vi "Sequence Execution.vi"() -> ()   [LabVIEW 2013, in "Simple Sequence Tools - Execution.lvlib"]
uses:
  Simple Sequence Tools - Execution.lvlib
  Types/Execute.PreviewMode.ctl
  Types/Execuction.StateVariables.ctl
  Types/Execute.UserEventRefs.ctl
  <vilib>/NI Veristand/Execution/Workspace/SystemStateRegEventRef.ctl
  Types/Execution.SequenceState.ctl
  <vilib>/NI Veristand/Execution/DataLogging/DataLoggingSpecification Ref.ctl
  <vilib>/NI Veristand/Execution/DataLogging/IDataLogging Ref.ctl
  <vilib>/NI Veristand/Execution/Workspace/WorkspaceAPI.ctl
  <vilib>/NI Veristand/Execution/Workspace/SystemStateEventRef.ctl
  Shared/Types/INI.Settings
  NationalInstruments.VeriStand.RealTimeSequenceDefinitionApi
  <vilib>/NI Veristand/Execution/Workspace/NI VeriStand - Set Single Channel Value.vi
  <vilib>/NI Veristand/Execution/Workspace/NI_VS Workspace ExecutionAPI.lvlib
  NationalInstruments.VeriStand.ClientAPI
  Shared/Simple Sequence Tools - Shared.lvlib
  <vilib>/NI Veristand/Execution/DataLogging/NI_VS Data Logging API.lvlib
panel:
  out "Total Iterations":u32=1 min=1 max=2
  out "Current Step":u32 min=1 max=5
  out "Current Iteration":u32=1 min=1 max=2
  in  "NIVS.Gateway IP Address":string="localhost"
  in  "NIVS.Workspace Event":refnum<event-registration>
  in  "Preview Mode":T1=enum."Table"
  in  "Start Step":u32 min=1 max=5
  in  "Start Iteration":u32=1 min=1 max=2
  in  "Log Channels":T2(ring)
  in  "Base File Name":string caption="Base File Name (timestamp included automatically)"
  in  "Enable Logging":bool
  in  "Abort":bool
  in  "Pause":bool
  in  "Start":bool
  in  "Profiles":string(combo)
  out "Graph":waveform(dbl)[](graph)
  out "Sequence":i32[](listbox)
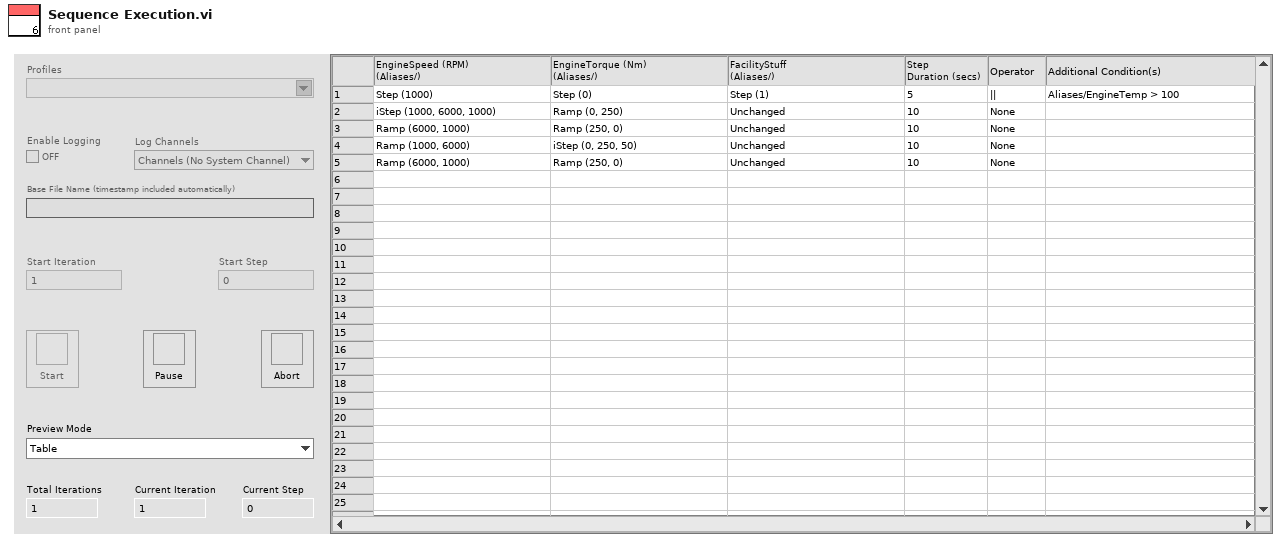
[diagram p1: front panel]
types:
  T1 = typedef "Simple Sequence Tools - Execution.lvlib/Execute.PreviewMode.ctl" = enum8{"Graph", "Table"}
  T2 = enum16{"Channels (No System Channel)", "Aliases", "All"}
  T3 = typedef "Simple Sequence Tools - Execution.lvlib/Execution.SequenceState.ctl" = enum16{"Idle", "Initializing", "Running", "Paused", "Finalizing", "Complete"}
  T4 = typedef "Simple Sequence Tools - Execution.lvlib/Execuction.StateVariables.ctl" = cluster{"NIVS.BaseLogPath":path, "NIVS.SystemDefinitionFile":path, "NIVS.Events":T5, "NIVS.SequenceState":T3, "NIVS.GatewayIPAddress":string, "NIVS.DataLogSpecRef":T7, "NIVS.DataLogManagerRef":T8, "NIVS.LogSessionGUID":string, "NIVS.WorkspaceManager":T9, "NIVS.Deployed":bool, "NIVS.ProfileRef":refnum<k24>, "NIVS.ProfileCallback":refnum<k27>, "NIVS.SystemStateRefs":T10, "UI.Abort":refnum<vi>, "UI.Pause":refnum<vi>, "UI.EnableLogging":refnum<vi>, "UI.Start":refnum<vi>, "UI.LogChannels":refnum<vi>, "UI.StartIteration":refnum<vi>, "UI.StartStep":refnum<vi>, "UI.Sequence":refnum<vi>, "UI.PreviewMode":refnum<vi>, "UI.Graph":refnum<vi>, "UI.BaseFileName":refnum<vi>, "UI.Profiles":refnum<vi>, "UI.CurrentStep":refnum<vi>, "UI.CurrentIteration":refnum<vi>, "UI.TotalIterations":refnum<vi>, "Sequence.AbortChannel":string, "Sequence.StepInfoChannel":string, "Sequence.Iterations":u32, "Sequence.IterationInfoChannel":string, "Sequence.#ofColumns":i32, "Events.State":refnum<user-event>, "Events.Test Result":refnum<user-event>, "Events.Progress":refnum<user-event>, "INI.Settings":T11}
  T5 = typedef "Simple Sequence Tools - Execution.lvlib/Execute.UserEventRefs.ctl" = cluster{"SequenceEvent":refnum<event-registration>, "SystemChangeEvent":T6, "WorkspaceEvent":refnum<event-registration>}
  T6 = typedef "NI_VS Workspace ExecutionAPI.lvlib/SystemStateRegEventRef.ctl" = refnum<event-registration>
  T7 = typedef "NI_VS Data Logging API.lvlib/DataLoggingSpecification Ref.ctl" = refnum<k24>
  T8 = typedef "NI_VS Data Logging API.lvlib/IDataLogging Ref.ctl" = refnum<k24>
  T9 = typedef "NI_VS Workspace ExecutionAPI.lvlib/WorkspaceAPI.ctl" = refnum<k24>
  T10 = typedef "NI_VS Workspace ExecutionAPI.lvlib/SystemStateEventRef.ctl" = cluster{"CustDatRef":refnum<user-event>, "EvtRef":refnum<k27>}
  T11 = typedef "Simple Sequence Tools - Shared.lvlib/INI.Settings" = cluster{"Build Location":path, "LoggingLocation":path}
  T12 = enum8{"Enabled", "Disabled", "Disabled and Grayed Out"}
  T13 = typedef "NI_VS Workspace ExecutionAPI.lvlib/SystemState.ctl" = u8
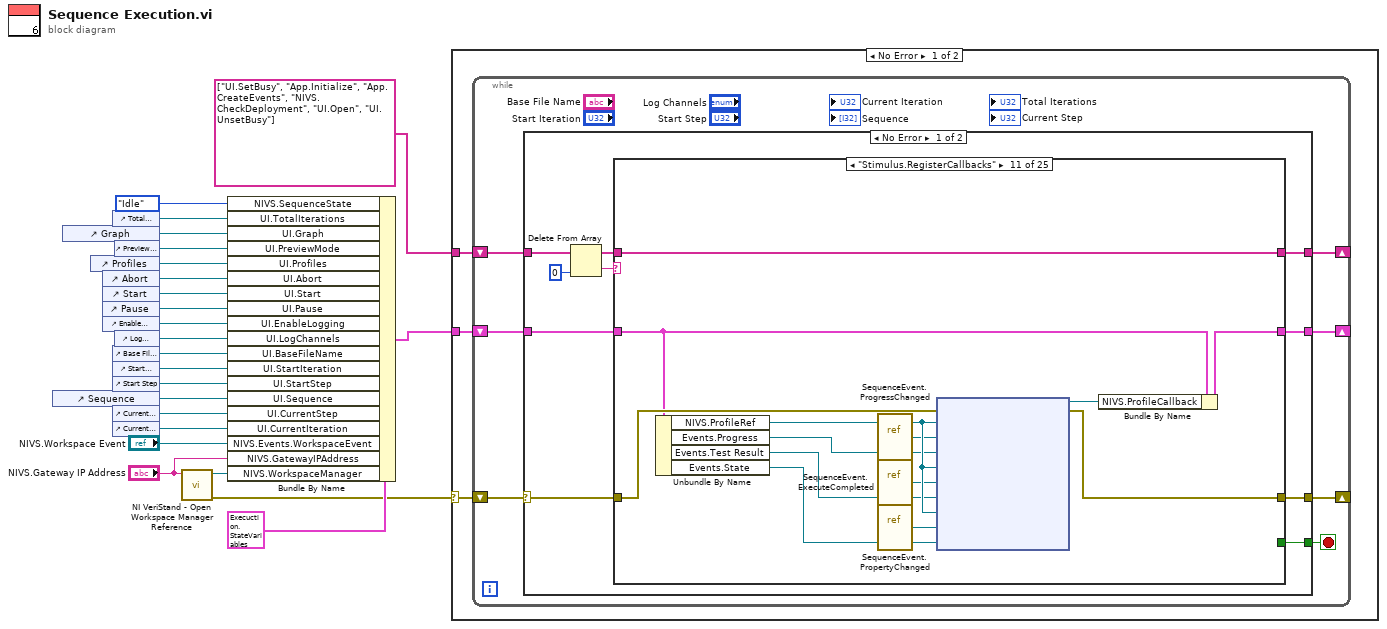
[diagram p0: block diagram]
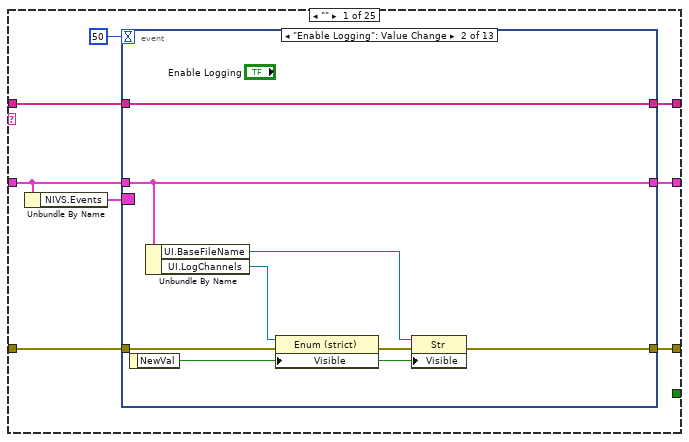
[diagram p2: hidden frame]
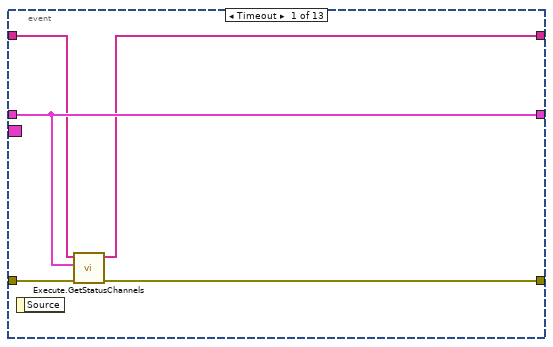
[diagram p3: hidden frame]
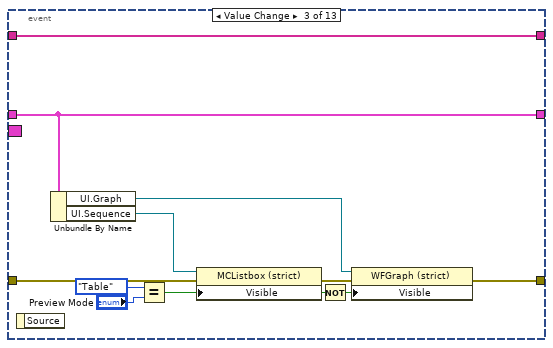
[diagram p4: hidden frame]
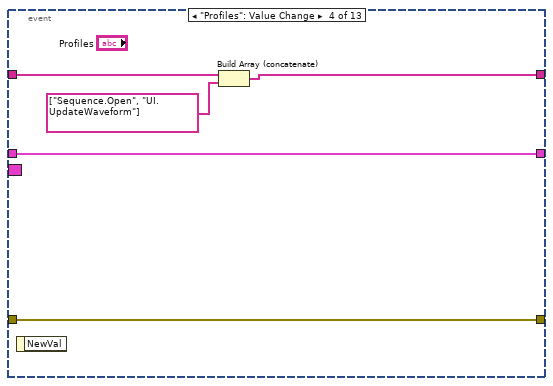
[diagram p5: hidden frame]
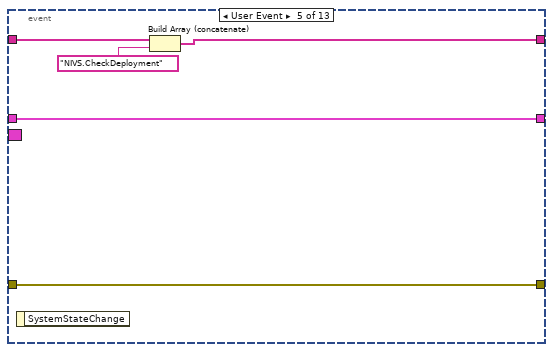
[diagram p6: hidden frame]
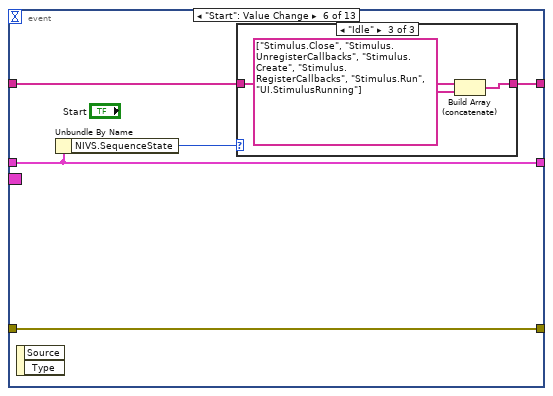
[diagram p7: hidden frame]
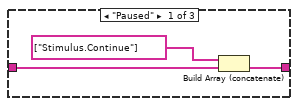
[diagram p8: hidden frame]
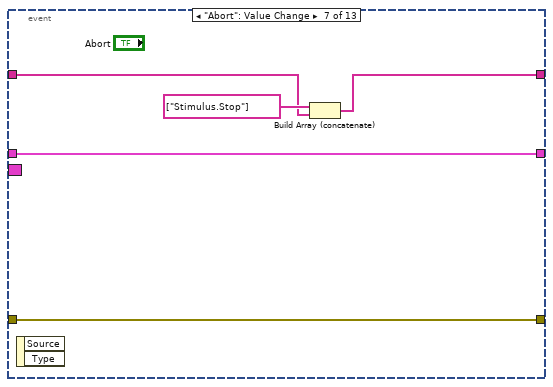
[diagram p10: hidden frame]
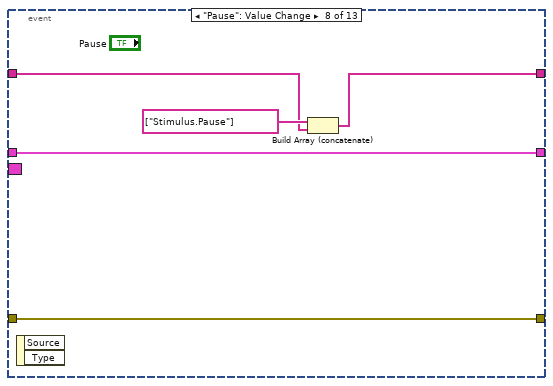
[diagram p11: hidden frame]
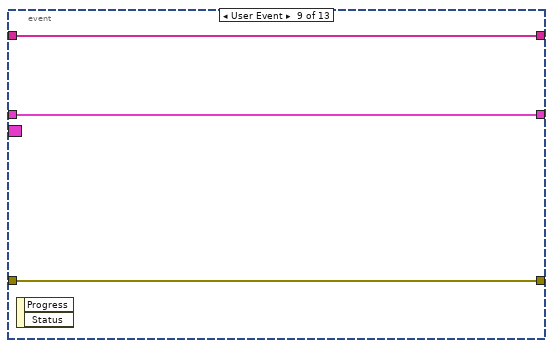
[diagram p12: hidden frame]
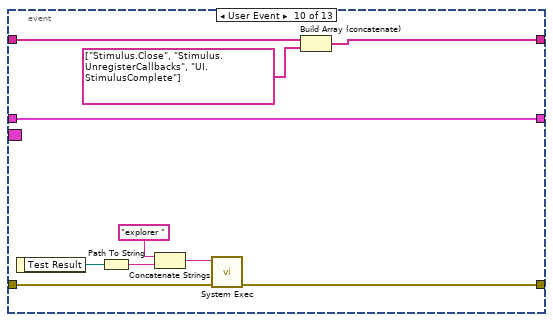
[diagram p13: hidden frame]
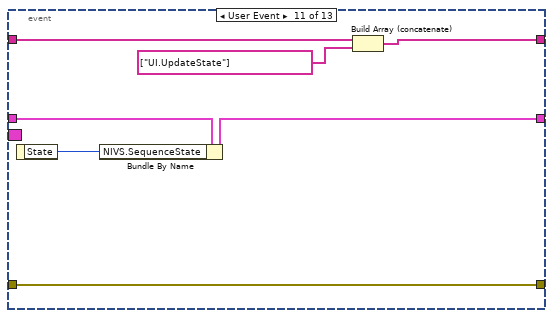
[diagram p14: hidden frame]
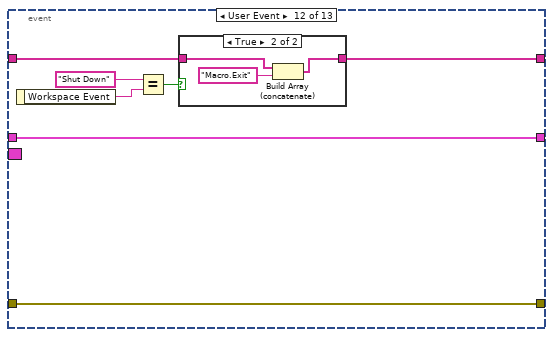
[diagram p15: hidden frame]
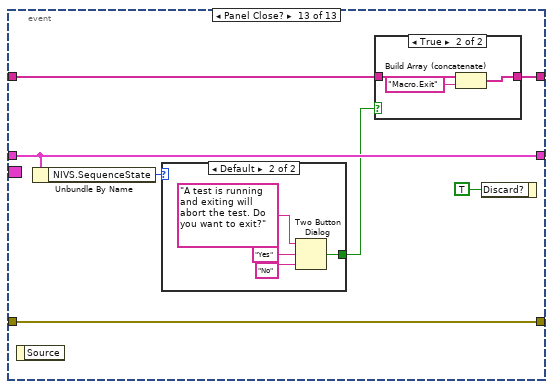
[diagram p17: hidden frame]
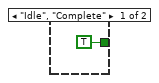
[diagram p19: hidden frame]
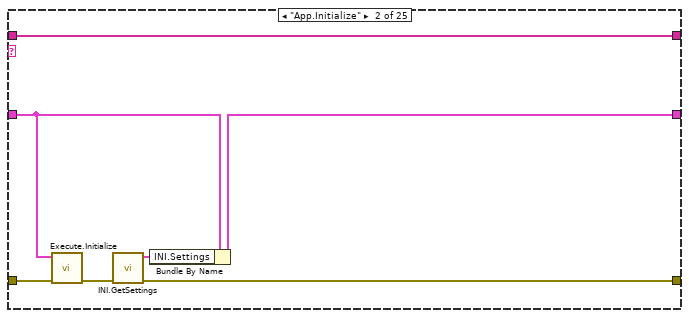
[diagram p20: hidden frame]
diagram:
  n1 = control-ref of="Sequence"() -> (w13:refnum<vi>)
  n2 = control-ref of="Graph"() -> (w22:refnum<vi>)
  n3 = control-ref of="Profiles"() -> (w11:refnum<vi>)
  n4 = control-ref of="Abort"() -> (w20:refnum<vi>)
  n5 = control-ref of="Start"() -> (w19:refnum<vi>)
  n6 = control-ref of="Pause"() -> (w18:refnum<vi>)
  n7 = control-ref of="Enable Logging"() -> (w17:refnum<vi>)
  n8 = control-ref of="Total Iterations"() -> (w4:refnum<vi>)
  n9 = control-ref of="Base File Name"() -> (w3:refnum<vi>)
  n10 = control-ref of="Start Iteration"() -> (w15:refnum<vi>)
  n11 = control-ref of="Start Step"() -> (w14:refnum<vi>)
  n12 = control-ref of="Current Step"() -> (w6:refnum<vi>)
  n13 = control-ref of="Current Iteration"() -> (w5:refnum<vi>)
  n14 = control-ref of="Preview Mode"() -> (w21:refnum<vi>)
  n15 = control-ref of="Log Channels"() -> (w16:refnum<vi>)
  n16 = call <vilib>:"NI VeriStand - Open Workspace Manager Reference.vi"("Gateway IP Address (\"\": localhost)"="NIVS.Gateway IP Address") -> ("error out"=w2:errorcluster, "WorkspaceManager"=w7:T9)  [unwired: 9 in]
  n17 = Bundle By Name(cluster=T4 {"NIVS.BaseLogPath"=path "", "NIVS.SystemDefinitionFile"=path "", "NIVS.Events"={"SequenceEvent"=refnum, "SystemChangeEvent"=refnum, "WorkspaceEvent"=refnum}, "NIVS.SequenceState"=enum."Idle", "NIVS.GatewayIPAddress"="", "NIVS.DataLogSpecRef"=refnum, "NIVS.DataLogManagerRef"=refnum, "NIVS.LogSessionGUID"="", "NIVS.WorkspaceManager"=refnum, "NIVS.Deployed"=FALSE, "NIVS.ProfileRef"=refnum, "NIVS.ProfileCallback"=refnum, "NIVS.SystemStateRefs"={"CustDatRef"=refnum, "EvtRef"=refnum}, "UI.Abort"=refnum, "UI.Pause"=refnum, "UI.EnableLogging"=refnum, "UI.Start"=refnum, "UI.LogChannels"=refnum, "UI.StartIteration"=refnum, "UI.StartStep"=refnum, "UI.Sequence"=refnum, "UI.PreviewMode"=refnum, "UI.Graph"=refnum, "UI.BaseFileName"=refnum, "UI.Profiles"=refnum, "UI.CurrentStep"=refnum, "UI.CurrentIteration"=refnum, "UI.TotalIterations"=refnum, "Sequence.AbortChannel"="", "Sequence.StepInfoChannel"="", "Sequence.Iterations"=0, "Sequence.IterationInfoChannel"="", "Sequence.#ofColumns"=0, "Events.State"=refnum, "Events.Test Result"=refnum, "Events.Progress"=refnum, "INI.Settings"={"Build Location"=path "", "LoggingLocation"=path ""}} ("Cluster"), "NIVS.SequenceState"=Execution.SequenceState."Idle", "UI.TotalIterations"=w4, "UI.Graph"=w22, "UI.PreviewMode"=w21, "UI.Profiles"=w11, "UI.Abort"=w20, "UI.Start"=w19, "UI.Pause"=w18, "UI.EnableLogging"=w17, "UI.LogChannels"=w16, "UI.BaseFileName"=w3, "UI.StartIteration"=w15, "UI.StartStep"=w14, "UI.Sequence"=w13, "UI.CurrentStep"=w6, "UI.CurrentIteration"=w5, "NIVS.Events.WorkspaceEvent"="NIVS.Workspace Event", "NIVS.GatewayIPAddress"="NIVS.Gateway IP Address", "NIVS.WorkspaceManager"=w7) -> (w12:T4)
  n18 = case shown="No Error" w2 {
    selector: w2 -> [w24 _]
    tunnel: string[] ["UI.SetBusy", "App.Initialize", "App.CreateEvents", "NIVS.CheckDeployment", "UI.Open", "UI.UnsetBusy"] -> [w26 _]
    tunnel: w12 -> [w25 w383]
    frame No Error {
      n19 = while {
        shift-right: [w32] -> _
        shift-left: w26 -> [w33]
        shift-right: [w30] -> _
        shift-left: w25 -> [w31]
        shift-right: [w28] -> _
        shift-left: w24 -> [w29]
        stop <- w27 stop-if-true
        n20 = case shown="No Error" w29 {
          selector: w29 -> [w34 w379]
          tunnel: w33 -> [w36 w382]
          tunnel: [w42 w382] -> w32
          tunnel: w31 -> [w40 w381]
          tunnel: [w39 w381] -> w30
          tunnel: [w38 w378] -> w28
          tunnel: [w37 _] -> w27
          frame No Error {
            n21 = Delete From Array(array=w36, index=0) -> (deleted portion=w43:string, array with subset deleted=w41:string[])  [unwired: 1 in]
            n22 = case shown="\"Stimulus.RegisterCallbacks\"" w43 {
              tunnel: [w49 w155 w166 w170 w171 w182 w186 w195 w229 w234 w247 w252 w258 w268 w280 w297 w308 w312 w315 w318 w322 w326 w339 w355 w377] -> w42
              tunnel: w41 -> [w48 w155 w166 w170 w171 w182 w187 w196 w229 w234 w247 w252 w258 w268 w280 w297 w308 w312 w315 w318 w322 w326 w339 w355 w377]
              tunnel: w40 -> [w45 w156 w162 w167 w177 w183 w189 w198 w226 w231 w238 w249 w257 w267 w277 w299 w306 w311 w314 w317 w319 w323 w338 w349 w376]
              tunnel: [w51 w159 w164 w167 w177 w183 w189 w197 w225 w230 w239 w248 w257 w267 w277 w299 w306 w311 w314 w317 w319 w323 w338 w349 w376] -> w39
              tunnel: [w46 w160 w165 w168 w181 w185 w190 w193 w227 w232 w245 w251 w253 w263 w278 w296 w307 w309 w313 w316 w320 w324 w332 w353 w375] -> w38
              tunnel: w34 -> [w47 w161 w163 w169 w181 w185 w190 w194 w228 w233 w246 w250 w254 w264 w279 w296 w307 w310 w313 w316 w321 w325 w335 w354 w375]
              tunnel: [_ _ _ _ _ TRUE _ _ _ _ _ _ _ _ _ _ _ _ _ _ _ _ _ _ _] -> w37
              frame "" {
                n23 = Unbundle By Name(w45) -> ("NIVS.Events"=w44:T5)
                n24 = event shown="[1] \"Enable Logging\": Value Change" {
                  selector: w44 -> [_ _ _ _ _ _ _ _ _ _ _ _ _]
                  dyn-events: _ -> [_ _ _ _ _ _ _ _ _ _ _ _ _]
                  timeout: 50 -> [_ _ _ _ _ _ _ _ _ _ _ _ _]
                  tunnel: [w53 w64 w75 w79 w84 w88 w98 w103 w110 w118 w121 w129 w142] -> w49
                  tunnel: w48 -> [w54 w64 w75 w80 w85 w89 w99 w104 w110 w119 w122 w132 w145]
                  tunnel: [w56 w63 w72 w78 w82 w87 w102 w107 w109 w120 w124 w134 w141] -> w51
                  tunnel: w45 -> [w56 w63 w72 w78 w82 w87 w102 w107 w109 w120 w125 w134 w141]
                  tunnel: [w52 w57 w65 w77 w81 w90 w101 w106 w108 w115 w127 w133 w144] -> w46
                  tunnel: w47 -> [w55 w61 w66 w77 w81 w90 w101 w106 w108 w116 w127 w133 w144]
                  event Timeout {
                    n25 = event-data() -> ()  [unwired: 1 in, 1 out]
                    n26 = call "Execute.GetStatusChannels.vi"("error in (no error)"=w55, "Cluster"=w56, "Commands"=w54) -> ("error out"=w52:errorcluster, "Commands out"=w53:string[])  [unwired: 7 in]
                  }
                  event "Enable Logging": Value Change {
                    n27 = event-data() -> ("NewVal"=w58:bool)  [unwired: 1 in]
                    n28 = Unbundle By Name(w63) -> ("UI.BaseFileName"=w59:refnum<vi>, "UI.LogChannels"=w62:refnum<vi>)
                    n29 = property class="Enum (strict)"(reference=w62, error in=w61, "Visible"=w58) -> (error out=w60:errorcluster)  [unwired: 1 out]
                    n30 = property class="Str"(reference=w59, error in=w60, "Visible"=w58) -> (error out=w57:errorcluster)  [unwired: 1 out]
                  }
                  event Value Change {
                    n31 = event-data() -> ()  [unwired: 1 in, 1 out]
                    n32 = Unbundle By Name(w72) -> ("UI.Graph"=w70:refnum<vi>, "UI.Sequence"=w71:refnum<vi>)
                    n33 = Equal?(x=Execute.PreviewMode."Table" ("y"), y="Preview Mode") -> (x = y?=w68:bool)
                    n34 = property class="MCListbox (strict)"(reference=w71, error in=w66, "Visible"=w68) -> (error out=w69:errorcluster)  [unwired: 1 out]
                    n35 = Not(x=w68) -> (.not. x?=w67:bool)
                    n36 = property class="WFGraph (strict)"(reference=w70, error in=w69, "Visible"=w67) -> (error out=w65:errorcluster)  [unwired: 1 out]
                  }
                  event "Profiles": Value Change {
                    n37 = event-data() -> ()  [unwired: 1 in, 1 out]
                    n38 = Build Array (concatenate)(w80, string[] ["Sequence.Open", "UI.UpdateWaveform"]) -> (w79:string[])
                  }
                  event User Event {
                    n39 = event-data() -> ()  [unwired: 1 in, 1 out]
                    n40 = Build Array (concatenate)(w85, "NIVS.CheckDeployment") -> (w84:string[])
                  }
                  event "Start": Value Change {
                    n41 = event-data() -> ()  [unwired: 1 in, 2 out]
                    n42 = Unbundle By Name(w87) -> ("NIVS.SequenceState"=w86:T3)
                    n43 = case shown="\"Idle\"" w86 {
                      tunnel: w89 -> [w92 w94 w97]
                      tunnel: [w91 w94 w96] -> w88
                      frame "Paused" {
                        n44 = Build Array (concatenate)(string[] ["Stimulus.Continue"] ("array"), w92) -> (w91:string[])
                      }
                      frame Default {
                      }
                      frame "Idle" {
                        n45 = Build Array (concatenate)(w97, string[] ["Stimulus.Close", "Stimulus.UnregisterCallbacks", "Stimulus.Create", "Stimulus.RegisterCallbacks", "Stimulus.Run", "UI.StimulusRunning"] ("array")) -> (w96:string[])
                      }
                    }
                  }
                  event "Abort": Value Change {
                    n46 = event-data() -> ()  [unwired: 1 in, 2 out]
                    n47 = Build Array (concatenate)(string[] ["Stimulus.Stop"] ("array"), w99) -> (w98:string[])
                  }
                  event "Pause": Value Change {
                    n48 = event-data() -> ()  [unwired: 1 in, 2 out]
                    n49 = Build Array (concatenate)(string[] ["Stimulus.Pause"] ("array"), w104) -> (w103:string[])
                  }
                  event User Event {
                    n50 = event-data() -> ()  [unwired: 1 in, 2 out]
                  }
                  event User Event {
                    n51 = event-data() -> ("Test Result"=w114:path)  [unwired: 1 in]
                    n52 = Path To String(path=w114) -> (string=w113:string)
                    n53 = Concatenate Strings("explorer " ("string"), w113) -> (w112:string)
                    n54 = call <vilib>:"System Exec.vi"("error in (no error)"=w116, "command line"=w112) -> ("error out"=w115:errorcluster)  [unwired: 6 in, 3 out]
                    n55 = Build Array (concatenate)(w119, string[] ["Stimulus.Close", "Stimulus.UnregisterCallbacks", "UI.StimulusComplete"]) -> (w118:string[])
                  }
                  event User Event {
                    n56 = event-data() -> ("State"=w126:i32)  [unwired: 1 in]
                    n57 = Bundle By Name(cluster=w125, "NIVS.SequenceState"=w126) -> (w124:T4)
                    n58 = Build Array (concatenate)(w122, string[] ["UI.UpdateState"] ("array")) -> (w121:string[])
                  }
                  event User Event {
                    n59 = event-data() -> ("Workspace Event"=w128:string)  [unwired: 1 in]
                    n60 = Equal?(x="Shut Down" ("y"), y=w128) -> (x = y?=w130:bool)
                    n61 = case shown="True" w130 {
                      tunnel: w132 -> [w135 w138]
                      tunnel: [w135 w136] -> w129
                      frame False {
                      }
                      frame True {
                        n62 = Build Array (concatenate)(w138, "Macro.Exit" ("y")) -> (w136:string[])
                      }
                    }
                  }
                  event Panel Close? {
                    n63 = event-data() -> ()  [unwired: 1 in, 1 out]
                    n64 = Unbundle By Name(w141) -> ("NIVS.SequenceState"=w140:T3)
                    n65 = case shown="Default" w140 {
                      tunnel: [TRUE ("T button?") w151] -> w139
                      frame "Idle", "Complete" {
                      }
                      frame Default {
                        n66 = Two Button Dialog(message="A test is running and exiting will abort the test. Do you want to exit?", 1:"No" ("F button name (\"Cancel\")"), 2:"Yes" ("T button name (\"OK\")")) -> (T button?=w151:bool)
                      }
                    }
                    n67 = case shown="True" w139 {
                      tunnel: w145 -> [w146 w149]
                      tunnel: [w146 w148] -> w142
                      frame False {
                      }
                      frame True {
                        n68 = Build Array (concatenate)(w149, "Macro.Exit") -> (w148:string[])
                      }
                    }
                    n69 = event-data("Discard?"=TRUE) -> ()  [unwired: 1 in, 1 out]
                  }
                }
              }
              frame "App.Initialize" {
                n70 = call "Execute.Initialize.vi"("error in (no error)"=w161, "Cluster"=w156) -> ("error out"=w157:errorcluster)  [unwired: 9 in]
                n71 = call "INI.GetSettings.vi"("error in (no error)"=w157) -> ("error out"=w160:errorcluster, "INI.Settings"=w158:T11)  [unwired: 9 in]
                n72 = Bundle By Name(cluster=w156, "INI.Settings"=w158) -> (w159:T4)
              }
              frame "App.CreateEvents" {
                n73 = call "Execute.CreateEvents.vi"("error in (no error)"=w163, "Cluster in"=w162) -> ("error out"=w165:errorcluster, "Cluster out"=w164:T4)  [unwired: 8 in]
              }
              frame "App.LoadSequences" {
                n74 = call "Execute.LoadSequences.vi"("error in (no error)"=w169, "Cluster"=w167) -> ("error out"=w168:errorcluster)  [unwired: 9 in]
              }
              frame "App.CloseReferences" {
                n75 = Unbundle By Name(w177) -> ("NIVS.Events.WorkspaceEvent"=w173:refnum<event-registration>, "Events.State"=w178:refnum<user-event>, "Events.Test Result"=w179:refnum<user-event>, "Events.Progress"=w180:refnum<user-event>, "NIVS.Events"=w176:T5, "NIVS.SystemStateRefs"=w175:T10, "NIVS.WorkspaceManager"=w174:T9)
                n76 = call <vilib>:"NI VeriStand - Close Workspace Manager Reference.vi"("WorkspaceManager"=w174) -> ()  [unwired: 10 in, 1 out]
                n77 = call <vilib>:"NI VeriStand - Close Engine State Change Notification.vi"("SystemStateRefs"=w175) -> ()  [unwired: 10 in, 1 out]
                n78 = Unregister For Events(event registration refnum=w176) -> ()  [unwired: 1 in, 1 out]
                n79 = Destroy User Event(user event=w180) -> ()  [unwired: 1 in, 1 out]
                n80 = Destroy User Event(user event=w179) -> ()  [unwired: 1 in, 1 out]
                n81 = Destroy User Event(user event=w178) -> ()  [unwired: 1 in, 1 out]
                n82 = Not A Number/Path/Refnum?(number/path/refnum=w173) -> (NaN/Path/Refnum?=w172:bool)
                n83 = case shown="False" w172 {
                  frame False {
                    n84 = invoke class="VI" method="FP.Close"() -> ()  [unwired: 3 in, 3 out]
                  }
                  frame True {
                  }
                }
              }
              frame "App.Exit" {
              }
              frame "Macro.Exit" {
                n85 = Build Array (concatenate)(w187, string[] ["Stimulus.Stop", "Stimulus.Close", "Stimulus.UnregisterCallbacks", "App.CloseReferences", "App.Exit"]) -> (w186:string[])
              }
              frame "NIVS.CheckDeployment" {
                n86 = Unbundle By Name(w198) -> ("INI.Settings.LoggingLocation"=w192:path, "NIVS.WorkspaceManager"=w199:T9)
                n87 = call <vilib>:"NI VeriStand - Get System State.vi"("error in (no error)"=w194, "WorkspaceManager in"=w199) -> ("error out"=w193:errorcluster, "System State"=w200:T13, "System Definition File"=w191:path)  [unwired: 5 in, 2 out]
                n88 = case shown="1" w200 {
                  tunnel: w196 -> [w204 w218]
                  tunnel: [w203 w217] -> w195
                  tunnel: w198 -> [w207 w215]
                  tunnel: [w206 w213] -> w197
                  tunnel: w192 -> [_ w210]
                  tunnel: w191 -> [_ w209]
                  frame 0, Default {
                    w201 = path ""
                    # "Not connected"
                    n89 = Bundle By Name(cluster=w207, "NIVS.Deployed"=FALSE ("Connected"), "NIVS.SystemDefinitionFile"=w201, "NIVS.BaseLogPath"=w201) -> (w206:T4)
                    n90 = Build Array (concatenate)(w204, "App.Initialize") -> (w203:string[])
                  }
                  frame 1 {
                    # "Connected"
                    n91 = Empty String/Path?(string/path=w210) -> (empty?=w211:bool)
                    n92 = case shown="True" w211 {
                      tunnel: [w220 w222] -> w212
                      tunnel: w210 -> [w220 _]
                      tunnel: w209 -> [w219 w221]
                      tunnel: [w219 w221] -> w208
                      frame False {
                      }
                      frame True {
                        n93 = Strip Path(path=w221) -> (stripped path=w224:path)  [unwired: 1 out]
                        n94 = Build Path(base path=w224, name or relative path="Logs") -> (appended path=w222:path)
                      }
                    }
                    n95 = Build Array (concatenate)(string[] ["App.LoadSequences", "UI.Connected"], w218) -> (w217:string[])
                    n96 = Bundle By Name(cluster=w215, "NIVS.Deployed"=TRUE ("Connected"), "NIVS.BaseLogPath"=w212, "NIVS.SystemDefinitionFile"=w208) -> (w213:T4)
                  }
                }
              }
              frame "Sequence.Open" {
                n97 = call "Execute.InitializeSequence.vi"("error in (no error)"=w228, "State Variables"=w226) -> ("error out"=w227:errorcluster, "State Variables"=w225:T4)  [unwired: 8 in]
              }
              frame "Stimulus.Create" {
                n98 = call "Execute.RunStimulus.vi"("error in (no error)"=w233, "State Variables"=w231) -> ("error out"=w232:errorcluster, "State Variables"=w230:T4)  [unwired: 8 in]
              }
              frame "Stimulus.RegisterCallbacks" {
                n99 = Unbundle By Name(w238) -> ("NIVS.ProfileRef"=w244:refnum<k24>, "Events.Progress"=w243:refnum<user-event>, "Events.Test Result"=w242:refnum<user-event>, "Events.State"=w241:refnum<user-event>)
                n100 = vi-ref "SequenceEvent.ProgressChanged.vi"() -> ("vi reference"=w237:refnum<vi>)
                n101 = vi-ref "SequenceEvent.ExecuteCompleted.vi"() -> ("vi reference"=w236:refnum<vi>)
                n102 = vi-ref "SequenceEvent.PropertyChanged.vi"() -> ("vi reference"=w235:refnum<vi>)
                n103 = node(w246, w244, w237, w243, w244, w236, w242, w244, w235, w241) -> (w240:refnum<k27>, w245:errorcluster)  [unwired: 1 in]
                n104 = Bundle By Name(cluster=w238, "NIVS.ProfileCallback"=w240) -> (w239:T4)
              }
              frame "Stimulus.Run" {
                n105 = call "Execute.Stimulus.Run.vi"("error in (no error)"=w250, "Cluster in"=w249) -> ("error out"=w251:errorcluster, "Cluster out"=w248:T4)  [unwired: 8 in]
              }
              frame "Stimulus.Pause" {
                n106 = Unbundle By Name(w257) -> ("NIVS.SequenceState"=w255:T3, "NIVS.ProfileRef"=w256:refnum<k24>)
                n107 = case shown="\"Running\"" w255 {
                  tunnel: w256 -> [_ w262]
                  tunnel: w254 -> [w259 w261]
                  tunnel: [w259 w260] -> w253
                  frame "Idle", Default {
                  }
                  frame "Running" {
                    n108 = invoke class="StimulusProfile" method="Pause"(reference=w262, error in=w261) -> (error out=w260:errorcluster)  [unwired: 1 in, 2 out]
                  }
                }
              }
              frame "Stimulus.Continue" {
                n109 = Unbundle By Name(w267) -> ("NIVS.SequenceState"=w266:T3, "NIVS.ProfileRef"=w265:refnum<k24>)
                n110 = case shown="\"Paused\"" w266 {
                  tunnel: w265 -> [_ w272]
                  tunnel: w264 -> [w269 w271]
                  tunnel: [w269 w270] -> w263
                  frame "Idle", Default {
                  }
                  frame "Paused" {
                    n111 = invoke class="StimulusProfile" method="Continue"(reference=w272, error in=w271) -> (error out=w270:errorcluster)  [unwired: 1 in, 2 out]
                  }
                }
              }
              frame "Stimulus.Stop" {
                n112 = Unbundle By Name(w277) -> ("NIVS.WorkspaceManager"=w273:T9, "Sequence.AbortChannel"=w274:string, "NIVS.SequenceState"=w275:T3, "NIVS.ProfileRef"=w276:refnum<k24>)
                n113 = case shown="\"Running\", \"Paused\", Default" w275 {
                  tunnel: w276 -> [_ w283]
                  tunnel: w279 -> [w281 w287]
                  tunnel: [w281 w282] -> w278
                  tunnel: w274 -> [_ w286]
                  tunnel: w273 -> [_ w285]
                  frame "Idle" {
                  }
                  frame "Running", "Paused", Default {
                    n114 = case shown="Default" w286 {
                      selector: w286 -> [_ w290]
                      tunnel: w287 -> [w288 w293]
                      tunnel: [w288 w292] -> w284
                      tunnel: w285 -> [_ w291]
                      frame "" {
                      }
                      frame Default {
                        n115 = call-poly <vilib>:"NI VeriStand - Set Channel Value.vi"("error in (no error)"=w293, "Value"=1.0, "Channel"=w290, "WorkspaceManager in"=w291) -> ("error out"=w292:errorcluster)  [unwired: 6 in, 1 out]
                      }
                    }
                    n116 = invoke class="StimulusProfile" method="Stop"(reference=w283, error in=w284) -> (error out=w282:errorcluster)  [unwired: 1 in, 2 out]
                  }
                }
              }
              frame "Stimulus.Close" {
                n117 = Unbundle By Name(w299) -> ("NIVS.ProfileRef"=w298:refnum<k24>, "NIVS.DataLogManagerRef"=w295:T8, "NIVS.LogSessionGUID"=w294:string)
                n118 = case shown="Default" w294 {
                  selector: w294 -> [_ w301]
                  tunnel: w295 -> [_ w304]
                  tunnel: [_ w300] -> _
                  frame "" {
                  }
                  frame Default {
                    n119 = call <vilib>:"Stop Data Logging Session.vi"("Session Name in"=w301, "Data Logging Manager Ref in"=w304) -> ("error out"=w302:errorcluster, "Data Logging Manager Ref out"=w303:T8)  [unwired: 7 in, 1 out]
                    n120 = call <vilib>:"Close Data Logging Manager Reference.vi"("error in (no error)"=w302, "Data Logging Manager Ref in"=w303) -> ("error out"=w300:errorcluster)  [unwired: 9 in]
                  }
                }
                n121 = Close Reference(reference=w298) -> ()  [unwired: 1 in, 1 out]
              }
              frame "Stimulus.UnregisterCallbacks" {
                n122 = Unbundle By Name(w306) -> ("NIVS.ProfileCallback"=w305:refnum<k27>)
                n123 = Unregister For Events(event registration refnum=w305) -> ()  [unwired: 1 in, 1 out]
              }
              frame "UI.Open" {
                n124 = invoke class="VI" method="FP.Open"(error in=w310) -> (error out=w309:errorcluster)  [unwired: 4 in, 4 out]
              }
              frame "UI.SetBusy" {
                n125 = call <vilib>:"Set Busy.vi"() -> ()  [unwired: 10 in, 2 out]
              }
              frame "UI.UnsetBusy" {
                n126 = call <vilib>:"Unset Busy.vi"() -> ()  [unwired: 11 in, 1 out]
              }
              frame "UI.StimulusComplete" {
                n127 = call "Execute.UI.Complete.vi"("error in (no error)"=w321, "Cluster"=w319) -> ("error out"=w320:errorcluster)  [unwired: 9 in]
              }
              frame "UI.StimulusRunning" {
                n128 = call "Execute.UI.Running.vi"("error in (no error)"=w325, "Cluster"=w323) -> ("error out"=w324:errorcluster)  [unwired: 9 in]
              }
              frame "UI.UpdateState" {
                n129 = Unbundle By Name(w338) -> ("UI.Start"=w328:refnum<vi>, "UI.Abort"=w329:refnum<vi>, "UI.Pause"=w336:refnum<vi>, "NIVS.SequenceState"=w337:T3)
                n130 = case shown="\"Paused\"" w337 {
                  tunnel: [w341 w342 T12."Disabled and Grayed Out" ("Disabled") w346] -> w331
                  tunnel: [T12."Disabled and Grayed Out" ("Disabled") w342 w343 T12."Enabled" ("f")] -> w327
                  tunnel: [w341 w342 w343 w346] -> w330
                  frame "Running" {
                    w341 = T12."Enabled" ("Disabled")
                  }
                  frame Default {
                    w342 = T12."Disabled and Grayed Out" ("Disabled")
                  }
                  frame "Paused" {
                    w343 = T12."Enabled" ("Disabled")
                  }
                  frame "Idle" {
                    w346 = T12."Disabled and Grayed Out" ("Disabled")
                  }
                }
                n131 = property class="Bool"(reference=w336, error in=w335, "DisabledEnum"=w331) -> (error out=w334:errorcluster)  [unwired: 1 out]
                n132 = property class="Bool"(reference=w329, error in=w334, "DisabledEnum"=w330) -> (error out=w333:errorcluster)  [unwired: 1 out]
                n133 = property class="Bool"(reference=w328, error in=w333, "DisabledEnum"=w327) -> (error out=w332:errorcluster)  [unwired: 1 out]
              }
              frame "UI.UpdateWaveform" {
                n134 = Unbundle By Name(w349) -> ("NIVS.SequenceState"=w348:T3, "UI.Graph"=w350:refnum<vi>, "UI.Sequence"=w351:refnum<vi>, "Sequence.#ofColumns"=w352:i32)
                n135 = case shown="Default" w348 {
                  tunnel: w354 -> [w362 w369]
                  tunnel: [w361 w374] -> w353
                  tunnel: w352 -> [w359 w372]
                  tunnel: w351 -> [w358 w364]
                  tunnel: w350 -> [w357 w371]
                  tunnel: [w356 w370] -> w347
                  frame "Idle" {
                    n136 = call "Sequence.BuildPreviewWaveform.vi"("WaveformGraph in"=w357, "error in (no error)"=w362, "Rows"=cluster{"Start Index":i32, "Length":i32} {"Start Index"=0, "Length"=-1}, "UI.Sequence#ofColumns"=w359, "SequenceRef"=w358) -> ("error out"=w361:errorcluster, "Wavefrom"=w356:waveform(dbl)[])  [unwired: 5 in]
                  }
                  frame Default {
                    n137 = property class="MCListbox (strict)"(reference=w364, error in=w369) -> (reference out=w363:refnum<vi>, error out=w368:errorcluster, "Value"=w366:i32[])
                    n138 = Index Array(array=w366) -> (element=w365:i32)  [unwired: 1 in]
                    n139 = Bundle By Name(cluster=cluster{"Start Index":i32, "Length":i32} {"Start Index"=0, "Length"=1} ("Rows"), "Start Index"=w365) -> (w367:cluster{"Start Index":i32, "Length":i32})
                    n140 = call "Sequence.BuildPreviewWaveform.vi"("WaveformGraph in"=w371, "error in (no error)"=w368, "Rows"=w367, "UI.Sequence#ofColumns"=w372, "SequenceRef"=w363) -> ("error out"=w374:errorcluster, "Wavefrom"=w370:waveform(dbl)[])  [unwired: 5 in]
                  }
                }
                "Graph" <- w347
              }
              frame Default {
              }
            }
          }
          frame Error {
            n141 = call <vilib>:"Simple Error Handler.vi"("error in (no error)"=w379) -> ("error out"=w380:errorcluster)  [unwired: 4 in, 4 out]
            n142 = call <vilib>:"Clear Errors.vi"("error in (no error)"=w380) -> ("error out"=w378:errorcluster)  [unwired: 6 in]
          }
        }
      }
    }
    frame Error {
      n143 = Unbundle By Name(w383) -> ("NIVS.Events.WorkspaceEvent"=w385:refnum<event-registration>)
      n144 = Not A Number/Path/Refnum?(number/path/refnum=w385) -> (NaN/Path/Refnum?=w384:bool)
      n145 = case shown="False" w384 {
        frame False {
          n146 = invoke class="VI" method="FP.Close"() -> ()  [unwired: 3 in, 3 out]
        }
        frame True {
        }
      }
      n147 = One Button Dialog(message="NI VeriStand is not open. Please open NI VeriStand before running this utility.") -> ()  [unwired: 1 in, 1 out]
    }
  }
